vi "LVPortInvokeEvent.vi"(0 "ID":string, 1 "Category":string, 5 "name":string, 7 "Data":variant, 9 "Invoke? (t)":bool=TRUE, 11 "error in (no error)":errorcluster) -> (15 "error out":errorcluster)   [LabVIEW 2017]
uses:
  LVPortEventType.ctl
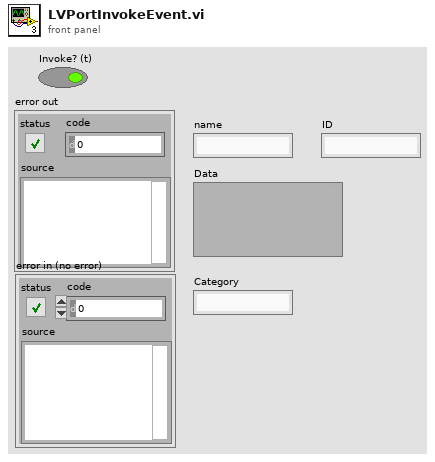
[diagram p1: front panel]
types:
  T1 = typedef "LVPortEventType.ctl" = cluster{"Name":string, "Data":variant}
  T2 = typedef "LVPortEventStreamDataType.ctl" = refnum<user-event>
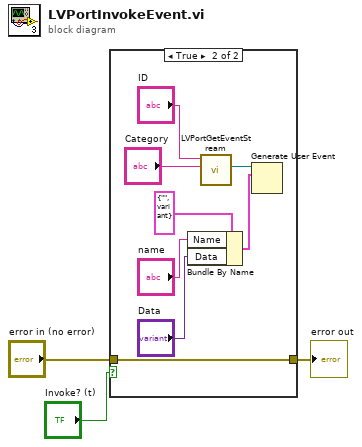
[diagram p0: block diagram]
diagram:
  n1 = case shown="True" "Invoke? (t)" {
    tunnel: "error in (no error)" -> [w4 w10]
    tunnel: [w4 w10] -> w1
    frame False {
    }
    frame True {
      n2 = Bundle By Name(cluster=T1 {"Name"="", "Data"=variant} ("event data"), "Name"="name", "Data"="Data") -> (w8:T1)
      n3 = call "LVPortGetEventStream.vi"("Category"="Category", "ID"="ID") -> ("EventStream"=w7:T2)  [unwired: 6 in, 3 out]
      n4 = Generate User Event(user event=w7, event data cluster=w8) -> ()  [unwired: 2 in, 2 out]
    }
  }
  "error out" <- w1
